vi "EnumToNIResolution.vi"(11 "Digit Resolution(5½)":T1) -> (3 "NI Resolution":dbl)   [LabVIEW 2020, in "NI DMM Driver.lvlib" / "DMM.NI.lvclass"]
doc: "Convert the Resolution Enum to a value the NI DMM can handle."
uses:
  DMM.NI.lvclass
  PPL/HDH.Driver.DMM.lvlibp/Controls/Ctl_DigitResolution.ctl
  PPL/HDH.Driver.DMM.lvlibp
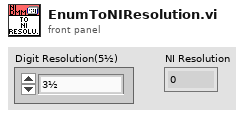
[diagram p1: front panel]
types:
  T1 = typedef "HDH.Driver.DMM.lvlibp/Ctl_DigitResolution.ctl" = enum8{"3½", "4½", "5½", "6½", "7½"}
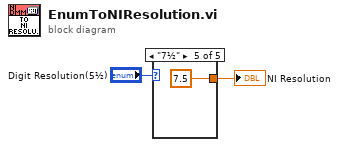
[diagram p0: block diagram]
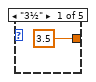
[diagram p2: hidden frame]
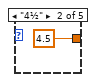
[diagram p3: hidden frame]
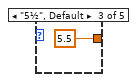
[diagram p4: hidden frame]
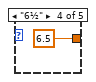
[diagram p5: hidden frame]
diagram:
  n1 = case shown="\"7½\"" "Digit Resolution(5½)" {
    tunnel: [3.5 ("Range") 4.5 ("Range") 5.5 ("Range") 6.5 ("Range") 7.5 ("Range")] -> w2
    frame "3½" {
    }
    frame "4½" {
    }
    frame "5½", Default {
    }
    frame "6½" {
    }
    frame "7½" {
    }
  }
  "NI Resolution" <- w2
